vi "Render Unescaped Tag.vi"(8 "Error In":errorcluster) -> (0 "Error Out":errorcluster)   [LabVIEW 2018, in "Tests.lvlib" / "Render.lvlib"]
uses:
  Render.lvlib
  src/Toolkit/Data/Map/Map.lvclass
  D:/Users/cfield/Code/Field R&D Services/Mustache/LabVIEW/trunk/src/Toolkit/Data/Abstract/Abstract.lvclass
  src/Toolkit/Low-Level/Support/Lex String.vi
  src/Toolkit/Data/Map/Support/From String.vi
  src/Toolkit/Low-Level/Support/Render to String.vi
  <vilib>/addons/_JKI Toolkits/Caraya/classes/Test/Test.lvclass
  <vilib>/addons/_JKI Toolkits/Caraya/classes/Assert/Assert.lvclass
  src/Toolkit/Toolkit.lvlib
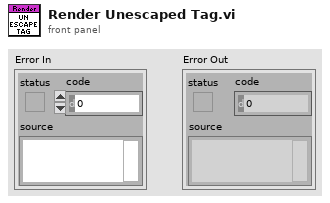
[diagram p1: front panel]
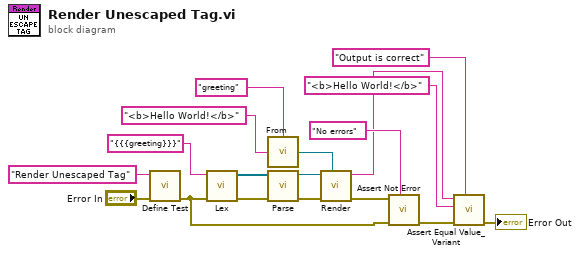
[diagram p0: block diagram]
diagram:
  n1 = call <vilib>:"Define Test.vi"("error in (no error)"="Error In", "Label (VI Title)"="Render Unescaped Tag") -> ("error out"=w1:errorcluster)  [unwired: 9 in]
  n2 = call-poly "Lex.vi"("Error In"=w1, "Input"="{{{greeting}}}" ("format string")) -> ("Error Out"=w10:errorcluster, "Tokens"=w8:refnum<class "Abstract.lvclass">[])  [unwired: 8 in]
  n3 = call-poly "From.vi"("Value"="<b>Hello World!</b>", "Key"="greeting") -> ("Map"=w2:refnum<class "Map.lvclass">)
  n4 = call "Parse.vi"("Error In"=w10, "Tokens"=w8) -> ("Error Out"=w7:errorcluster, "Abstract Syntax Tree"=w6:refnum<class "Root.lvclass">)  [unwired: 8 in]
  n5 = call-poly "Render.vi"("Data"=w2, "Error In"=w7, "Abstract Syntax Tree"=w6) -> ("Error Out"=w12:errorcluster, "Output"=w5:string)  [unwired: 7 in]
  n6 = call <vilib>:"Assert Not Error.vi"("Label"="No errors", "error in (no error)"=w1, "Not Error?"=w12) -> ("error out"=w15:errorcluster)  [unwired: 8 in]
  n7 = call <vilib>:"Assert Equal Value_Variant.vi"("Label"="Output is correct", "error in (no error)"=w15, "Y"="<b>Hello World!</b>" ("Value"), "X"=w5) -> ("error out"=→"Error Out":errorcluster)  [unwired: 7 in]
